vi "FTP Directory Creation.vi"(0 "Directory":string, 5 "Host":string, 7 "User":string="user", 9 "Password":string, 11 "error in (no error)":errorcluster) -> (4 "Directory Out":string, 6 "Standard Output":string, 15 "error out":errorcluster)   [LabVIEW 2011]
doc: "Use this VI to create an FTP Directory if it isn't created yet"
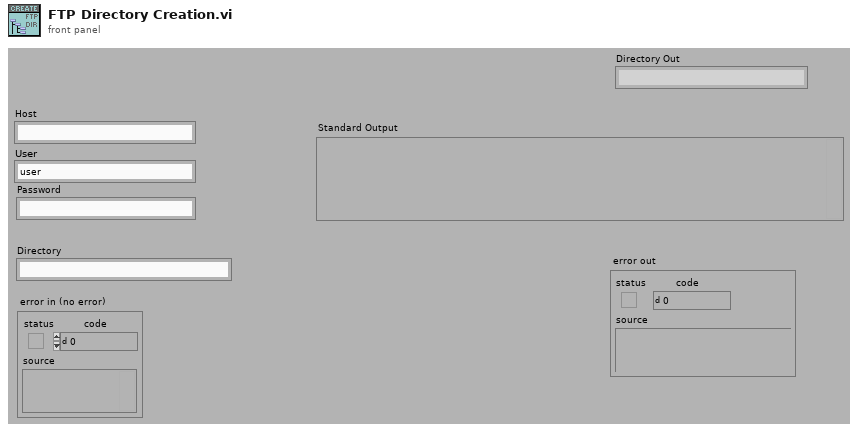
[diagram p1: front panel]
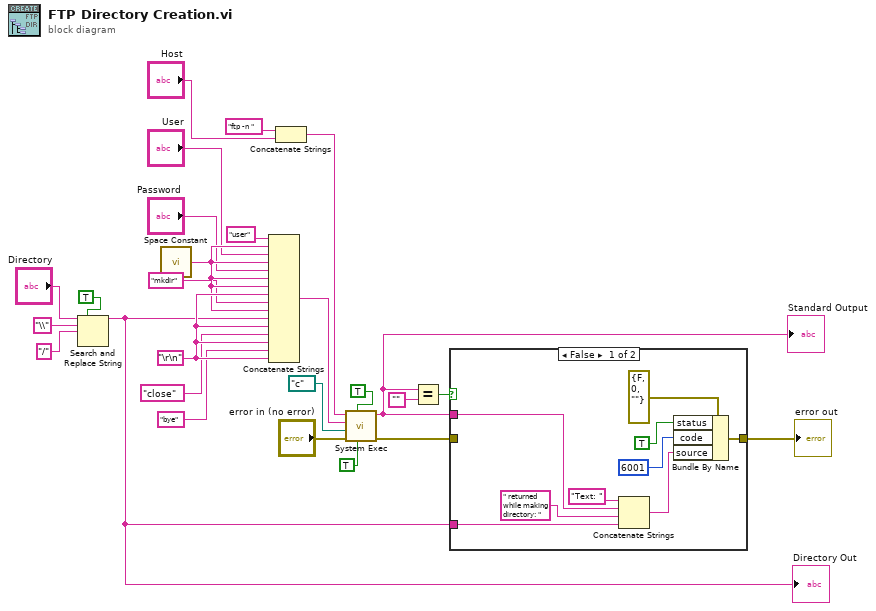
[diagram p0: block diagram]
diagram:
  w26 = "\r\n"
  n1 = Search and Replace String(replace all?=TRUE ("replace all? (F)"), input string="Directory", search string="\\", replace string="/" ("replace string (\"\")")) -> (result string=w22:string)  [unwired: 1 in, 6 out]
  "Directory Out" <- w22
  n2 = call <vilib>:"Space Constant.vi"() -> ("String"=w12:string)
  n3 = Concatenate Strings("user" ("string"), w12, "User", w12, "Password", w12, w12, w26, "mkdir" ("string"), w12, w22, w26, "close" ("string"), w26, "bye" ("string"), w26) -> (w4:string)
  n4 = Concatenate Strings("ftp -n " ("command line"), "Host") -> (w2:string)
  n5 = call <vilib>:"System Exec.vi"("run minimized? (F)"=TRUE, "wait until completion? (T)"=TRUE, "error in (no error)"="error in (no error)", "working directory"=path "c:/", "standard input"=w4, "command line"=w2) -> ("error out"=w19:errorcluster, "standard output"=w21:string)  [unwired: 4 out]
  "Standard Output" <- w21
  n6 = Equal?(x=w21, y="") -> (x = y?=w18:bool)
  n7 = case shown="False" w18 {
    tunnel: w19 -> [_ w36]
    tunnel: [w35 w36] -> w20
    tunnel: w21 -> [w30 _]
    tunnel: w22 -> [w28 _]
    frame False {
      n8 = Concatenate Strings("Text: ", w30, " returned while making directory: " ("string"), w28) -> (w27:string)
      n9 = Bundle By Name(cluster=errorcluster {"status"=FALSE, "code"=0, "source"=""} ("error out"), "status"=TRUE, "code"=6001, "source"=w27) -> (w35:errorcluster)
    }
    frame True {
    }
  }
  "error out" <- w20
